vi "Untitled 2.vi"() -> ()   [LabVIEW 2014]
uses:
  <vilib>/vision/NI_Vision_Development_Module.lvlib
  <vilib>/Utility/inputDevices.llb/keyboardAcquire.vi
panel:
  in  "填入飽和磁場分量尖點座標":dbl[][](array[numeric])
  in  "Stop Button":bool
  out "0. 原始畫面":T1(plugin-control)
  in  "1. 範圍選擇":T2={"色相（H）"={0, 255}, "飽和度（S）"={0, 255}, "亮度（L）"={0, 255}} {"亮度（L）" scale=0.0..255.0; "飽和度（S）" scale=0.0..255.0; "色相（H）" scale=0.0..255.0}
  in  "3. Number of Erosion":i32=10
  out "Number of Particles":i32
  out "output cluster":cluster{"X":dbl, "Y":dbl}
  in  "顏色範圍初始化":bool
  in  "Tab Control":T3(tab)
  out "1. 顏色選取":T1(plugin-control)
  out "2. 填補空隙":T1(plugin-control)
  out "3. 移除雜點":T1(plugin-control)
  out "4. 形狀修正":T1(plugin-control)
  out "5. 選取結果":T1(plugin-control)
  out "Particle Measurements":dbl[][](array[numeric])
  out "Error Out":errorcluster
  out "瞬間尖點座標":dbl[][](array[numeric])
  in  "停止":bool
  out "滑鼠位置顏色":T4
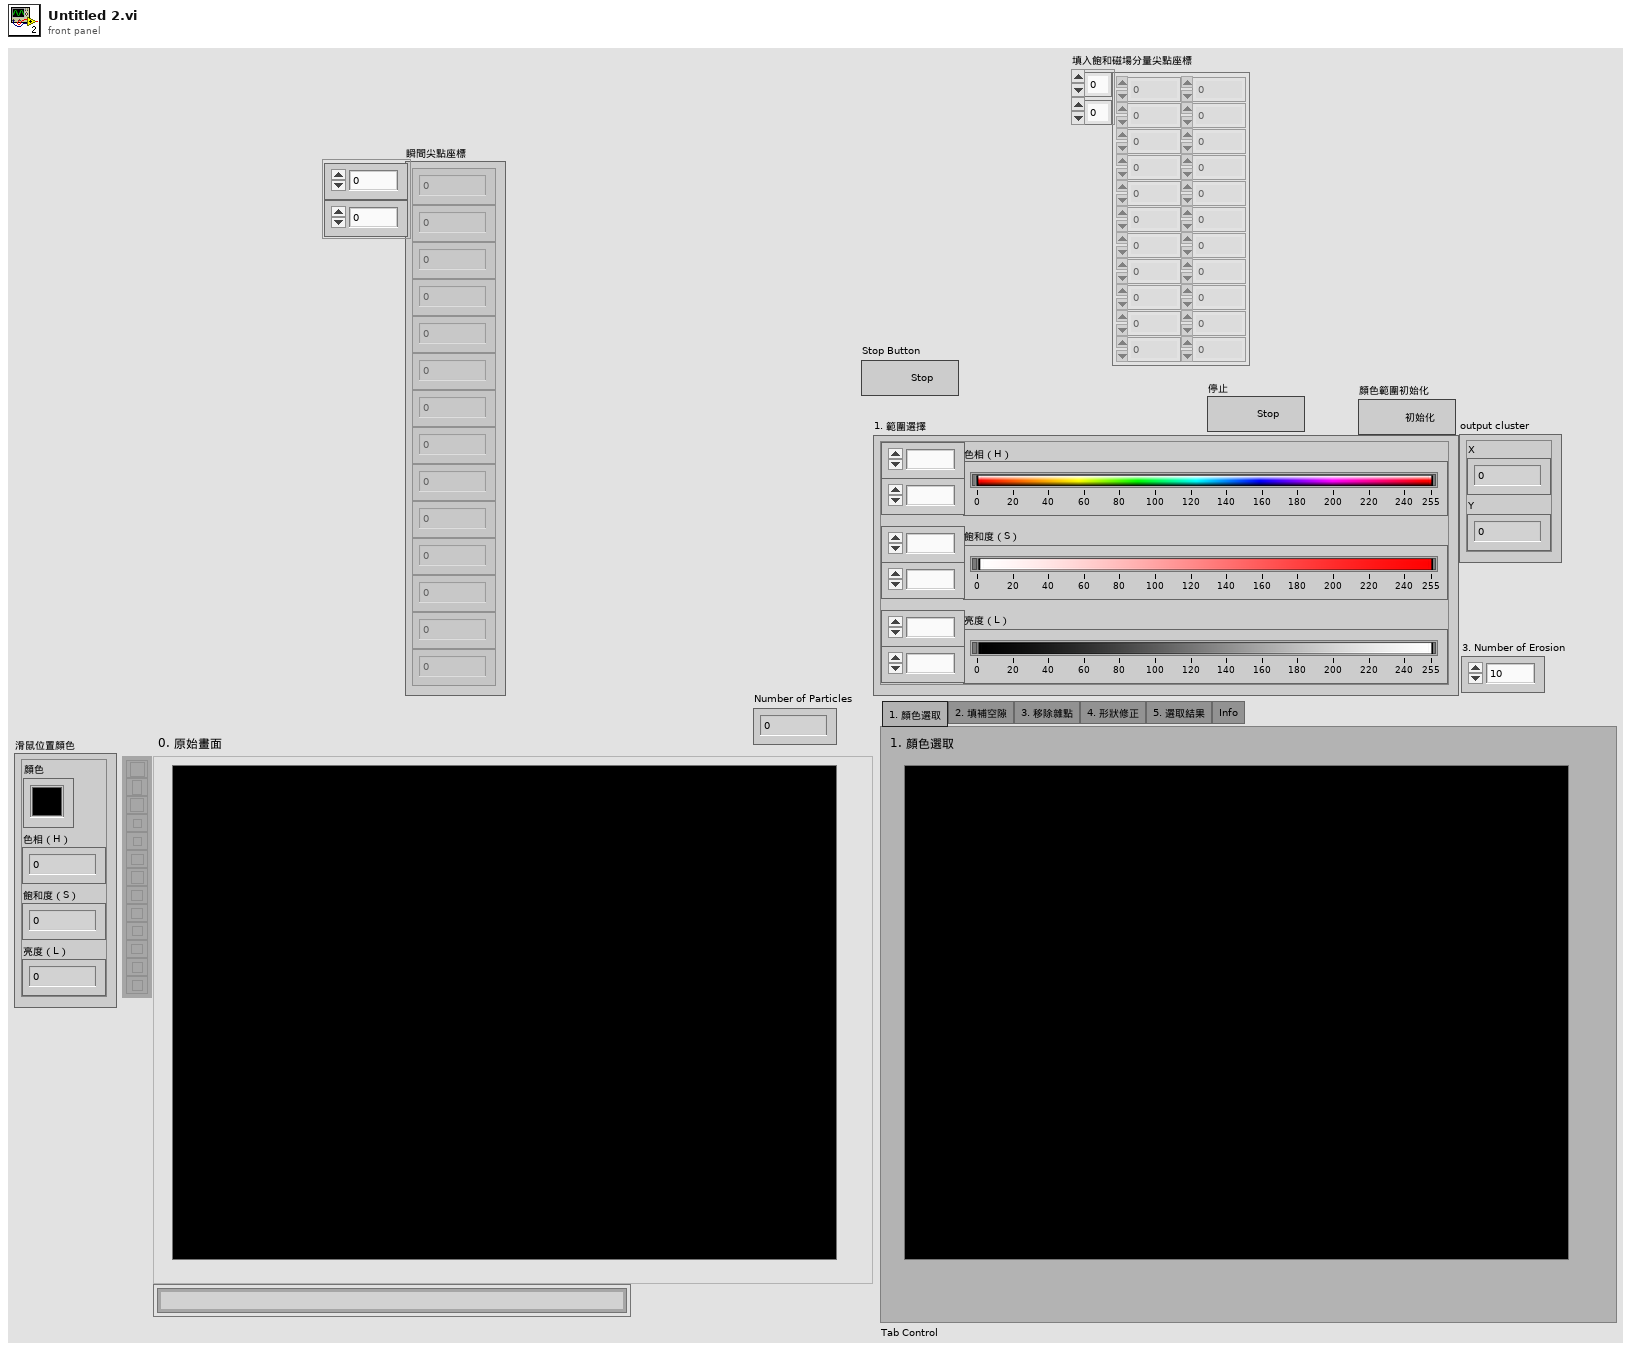
[diagram p1: front panel]
types:
  T1 = typedef "IMAQ Image.ctl" = refnum<image>
  T2 = cluster{"色相（H）":cluster{u8, u8}, "飽和度（S）":cluster{u8, u8}, "亮度（L）":cluster{u8, u8}}
  T3 = enum32{"1. 顏色選取", "2. 填補空隙", "3. 移除雜點", "4. 形狀修正", "5. 選取結果", "Info"}
  T4 = cluster{"色相（H）":u8, "飽和度（S）":u8, "亮度（L）":u8, "顏色":u32}
  T5 = enum16{"0", "1", "2", "3", "4", "5", "6", "7", "8", "9", "A", "B", "C", "D", "E", "F", "G", "H", "I", "J", "K", "L", "M", "N", "O", "P", "Q", "R", "S", "T", "U", "V", "W", "X", "Y", "Z", "F1", "F2", "F3", "F4", "F5", "F6", "F7", "F8", "F9", "F10", "F11", "F12", "F13", "F14", "F15", "ADD", "BACK", "BACKSLASH", "CAPITAL", "COMMA", "DECIMAL", "DELETE", "DIVIDE", "DOWN", "END", "EQUALS", "ESCAPE", "GRAVE (`)", "HOME", "INSERT", "LBRACKET", "LCONTROL", "LEFT", "L ALT", "LSHIFT", "LWIN", "MINUS", "MULTIPLY", "NEXT", "NUMLOCK", "NUMPAD_0", "NUMPAD_1", "NUMPAD_2", "NUMPAD_3", "NUMPAD_4", "NUMPAD_5", "NUMPAD_6", "NUMPAD_7", "NUMPAD_8", "NUMPAD_9", "PAUSE", "PERIOD", "PRIOR (PG UP)", "RBRACKET", "RCONTROL", "RETURN", "RIGHT", "R ALT", "RSHIFT", "RWIN", "SCROLL", "SEMICOLON", "SLASH", "SPACE", "SUBTRACT", "TAB", "UP", "ENTER (num pad)", "' (quote)"}[]
  T6 = enum16{"0", "1", "2", "3", "4", "5", "6", "7", "8", "9", "A", "B", "C", "D", "E", "F", "G", "H", "I", "J", "K", "L", "M", "N", "O", "P", "Q", "R", "S", "T", "U", "V", "W", "X", "Y", "Z", "F1", "F2", "F3", "F4", "F5", "F6", "F7", "F8", "F9", "F10", "F11", "F12", "F13", "F14", "F15", "ADD", "BACK", "BACKSLASH", "CAPITAL", "COMMA", "DECIMAL", "DELETE", "DIVIDE", "DOWN", "END", "EQUALS", "ESCAPE", "GRAVE (`)", "HOME", "INSERT", "LBRACKET", "LCONTROL", "LEFT", "L ALT", "LSHIFT", "LWIN", "MINUS", "MULTIPLY", "NEXT", "NUMLOCK", "NUMPAD_0", "NUMPAD_1", "NUMPAD_2", "NUMPAD_3", "NUMPAD_4", "NUMPAD_5", "NUMPAD_6", "NUMPAD_7", "NUMPAD_8", "NUMPAD_9", "PAUSE", "PERIOD", "PRIOR (PG UP)", "RBRACKET", "RCONTROL", "RETURN", "RIGHT", "R ALT", "RSHIFT", "RWIN", "SCROLL", "SEMICOLON", "SLASH", "SPACE", "SUBTRACT", "TAB", "UP", "ENTER (num pad)", "' (quote)"}
  T7 = cluster{"Numeric":dbl, "Numeric":dbl, "Numeric":dbl, "Numeric":dbl}
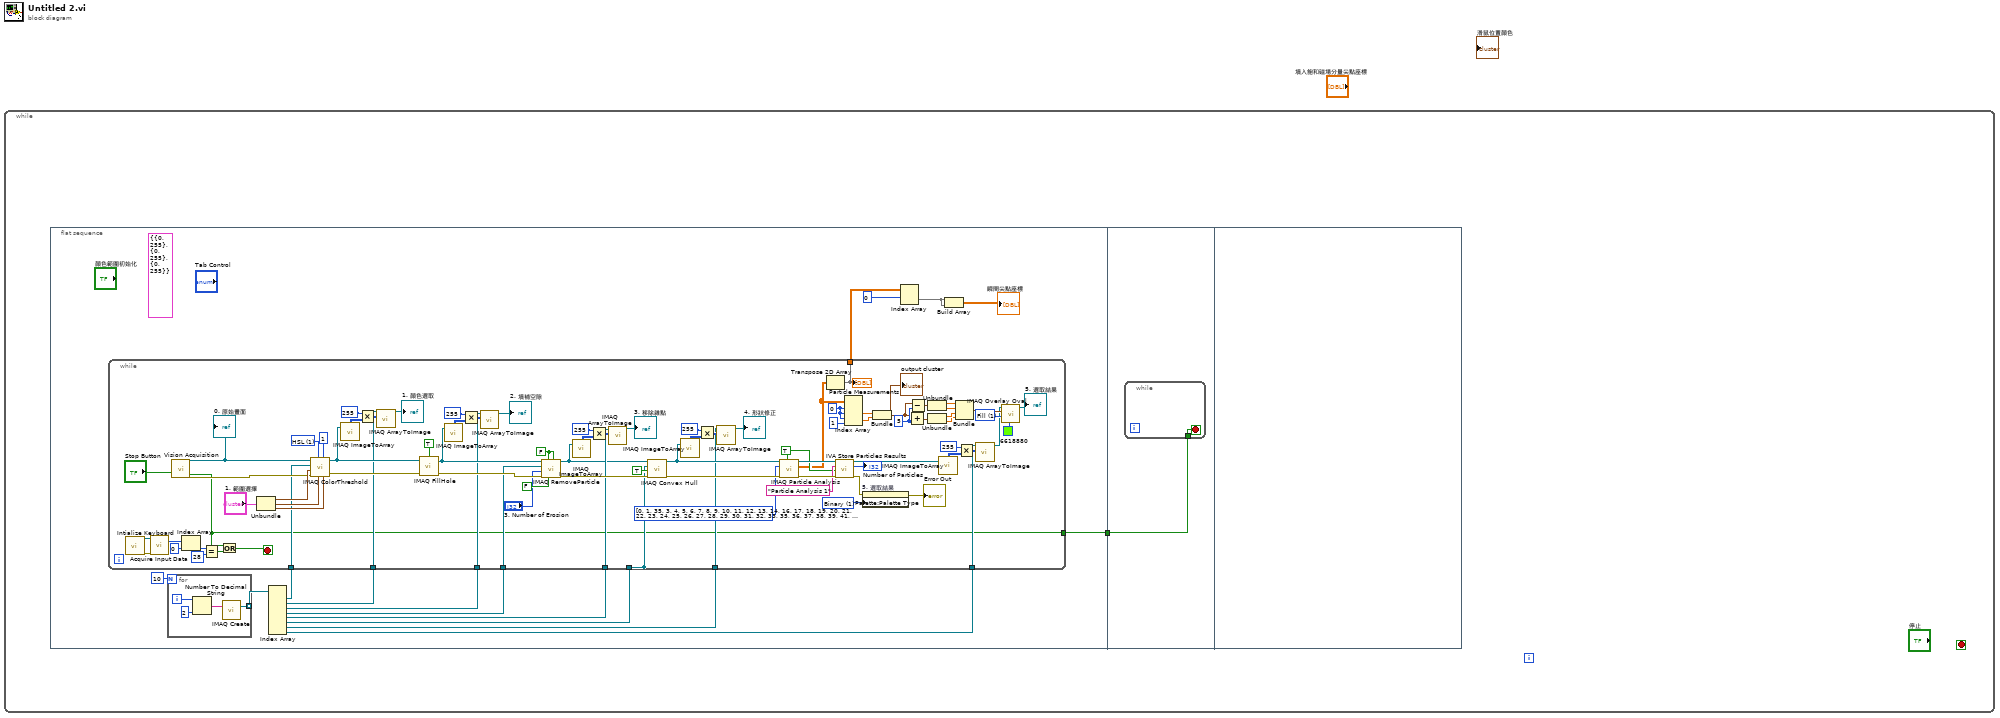
[diagram p0: block diagram]
diagram:
  n1 = while {
    stop <- _ stop-if-true
    n2 = flat-sequence {
      tunnel: [w2] -> w1
      tunnel: w1 -> [w108]
      frame #0 {
        (unwired) T2 {"色相（H）"={0, 255}, "飽和度（S）"={0, 255}, "亮度（L）"={0, 255}} ("範圍選擇")
        n3 = for {
          N: 10 -> [_]
          tunnel: [w17] -> w16 mode=indexing
          i -> [w19]
          n4 = Number To Decimal String(number=w19, width (-)=2) -> (decimal integer string=w18:string)
          n5 = call "IMAQ Create"("Image Name"=w18) -> ("New Image"=w17:T1)  [unwired: 4 in, 1 out]
        }
        n6 = Index Array(array=w16) -> (element #1=w15:T1, element #2=w14:T1, element #3=w13:T1, element #4=w11:T1, element #5=w10:T1, element #6=w9:T1, element #7=w8:T1, element #8=w7:T1)  [unwired: 8 in]
        n7 = while {
          tunnel: w13 -> [w62]
          tunnel: w11 -> [w77]
          tunnel: w9 -> [w75]
          tunnel: [w75] -> _
          tunnel: w14 -> [w69]
          tunnel: w15 -> [w61]
          tunnel: w10 -> [w57]
          tunnel: w8 -> [w49]
          tunnel: w7 -> [w27]
          tunnel: [w24] -> w5
          tunnel: [w21] -> w2
          stop <- w22 stop-if-true
          w32 = u32 1 items=["Frame", "Fill"] ("Drawing Mode (Frame)")
          w41 = 5
          w46 = 0
          w78 = u32 1 items=["Grayscale", "Binary", "Gradient", "Rainbow", "Temperature", "User Defined"] ("Palette")
          w87 = i32[] [0, 1, 35, 3, 4, 5, 6, 7, 8, 9, 10, 11, 12, 13, 14, 16, 17, 18, 19, 20, 21, 22, 23, 24, 25, 26, 27, 28, 29, 30, 31, 32, 33, 35, 36, 37, 38, 39, 41, 42, 43, 45, 46, 48, 49, 50, 51, 53, 54, 55, 56, 58, 59, 60, 61, 62, 63, 64, 65, 66, 68, 69, 70, 71, 72, 73, 74, 75, 76, 77, 78, 79, 80, 81, 82, 83, 84, 85, 86, 87, 88] items=["Center of Mass X", "Center of Mass Y", "First Pixel X", "First Pixel Y", "Bounding Rect Left", "Bounding Rect Top", "Bounding Rect Right", "Bounding Rect Bottom", "Max Feret Diameter Start X", "Max Feret Diameter Start Y", "Max Feret Diameter End X", "Max Feret Diameter End Y", "Max Horiz. Segment Length Left", "Max Horiz. Segment Length Right", "Max Horiz. Segment Length Row", "-", "Bounding Rect Width", "Bounding Rect Height", "Bounding Rect Diagonal", "Perimeter", "Convex Hull Perimeter", "Holes' Perimeter", "Max Feret Diameter", "Equivalent Ellipse Major Axis", "Equivalent Ellipse Minor Axis", "Equivalent Ellipse Minor Axis (Feret)", "Equivalent Rect Long Side", "Equivalent Rect Short Side", "Equivalent Rect Diagonal", "Equivalent Rect Short Side (Feret)", "Average Horiz. Segment Length", "Average Vert. Segment Length", "Hydraulic Radius", "Waddel Disk Diameter", "-", "Area", "Holes' Area", "Particle & Holes' Area", "Convex Hull Area", "Image Area", "-", "Number of Holes", "Number of Horiz. Segments", "Number of Vert. Segments", "-", "Orientation", "Max Feret Diameter Orientation", "-", "% Area/Image Area", "% Area/(Particle & Holes' Area)", "Ratio of Equivalent Ellipse Axes", "Ratio of Equivalent Rect Sides", "-", "Elongation Factor", "Compactness Factor", "Heywood Circularity Factor", "Type Factor", "-", "Sum X", "Sum Y", "Sum XX", "Sum XY", "Sum YY", "Sum XXX", "Sum XXY", "Sum XYY", "Sum YYY", "-", "Moment of Inertia XX", "Moment of Inertia XY", "Moment of Inertia YY", "Moment of Inertia XXX", "Moment of Inertia XXY", "Moment of Inertia XYY", "Moment of Inertia YYY", "Norm. Moment of Inertia XX", "Norm. Moment of Inertia XY", "Norm. Moment of Inertia YY", "Norm. Moment of Inertia XXX", "Norm. Moment of Inertia XXY", "Norm. Moment of Inertia XYY", "Norm. Moment of Inertia YYY", "Hu Moment 1", "Hu Moment 2", "Hu Moment 3", "Hu Moment 4", "Hu Moment 5", "Hu Moment 6", "Hu Moment 7"] ("Pixel Measurements")
          w89 = TRUE ("Connectivity 4/8 (8)")
          w68 = FALSE ("Connectivity 4/8 (8)")
          w98 = u16 1 items=["RGB", "HSL", "HSV", "HSI"] ("Color Mode")
          n8 = call <vilib>:"Intialize Keyboard.vi"() -> ("error out"=w102:errorcluster, "device ID"=w103:refnum<k1>)  [unwired: 10 in]
          n9 = call-poly <vilib>:"Acquire Input Data.vi"("device ID"=w103, "error in (no error)"=w102) -> ("keys pressed"=w104:T5)  [unwired: 15 in, 2 out]
          n10 = call "Vision Acquisition"("Stop (F)"="Stop Button") -> ("Image Out"=w100:T1, "Stopped"=w21:bool, "error out"=w93:errorcluster)  [unwired: 24 in]
          "0. 原始畫面" <- w100
          n11 = Index Array(array=w104, index=0) -> (element=w107:T6)
          n12 = Equal?(x=w107, y=28) -> (x = y?=w101:bool)
          n13 = Or(x=w21, y=w101) -> (x .or. y?=w22:bool)
          n14 = Unbundle("1. 範圍選擇") -> ("色相（H）"=w97:cluster{u8, u8}, "飽和度（S）"=w96:cluster{u8, u8}, "亮度（L）"=w95:cluster{u8, u8})
          n15 = call "IMAQ ColorThreshold"("Blue or Luma or Val or Inten Range"=w95, "Replace Value"=1, "Green or Sat Range"=w96, "Color Mode"=w98, "error in (no error)"=w93, "Red or Hue Range"=w97, "Image Dst"=w61, "Image Src"=w100) -> ("error out"=w80:errorcluster, "Image Dst Out"=w74:T1)  [unwired: 2 out]
          n16 = call "IMAQ ImageToArray"("Image"=w74) -> ("Image Pixels (U8)"=w72:u8[][])  [unwired: 3 in, 4 out]
          n17 = Multiply(x=255, y=w72) -> (x*y=w71:i32[][])
          n18 = call "IMAQ ArrayToImage"("Image Pixels (U8)"=w71, "Image"=w69) -> ("Image Out"=→"1. 顏色選取":T1)  [unwired: 8 in, 1 out]
          n19 = call "IMAQ FillHole"("error in (no error)"=w80, "Image Src"=w74, "Connectivity 4/8 (8)"=TRUE) -> ("error out"=w84:errorcluster, "Image Dst Out"=w63:T1)  [unwired: 1 in, 2 out]
          n20 = call "IMAQ ImageToArray"("Image"=w63) -> ("Image Pixels (U8)"=w66:u8[][])  [unwired: 3 in, 4 out]
          n21 = Multiply(x=255, y=w66) -> (x*y=w67:i32[][])
          n22 = call "IMAQ ArrayToImage"("Image Pixels (U8)"=w67, "Image"=w62) -> ("Image Out"=→"2. 填補空隙":T1)  [unwired: 8 in, 1 out]
          n23 = call "IMAQ RemoveParticle"("Connectivity 4/8 (8)"=w68, "Low Pass/High Pass (Low)"=FALSE, "Square/Hexa (Square)"=w68, "error in (no error)"=w84, "Number of Erosion"="3. Number of Erosion", "Image Dst"=w77, "Image Src"=w63) -> ("error out"=w85:errorcluster, "Image Dst Out"=w55:T1)  [unwired: 3 out]
          n24 = call "IMAQ ImageToArray"("Image"=w55) -> ("Image Pixels (U8)"=w59:u8[][])  [unwired: 3 in, 4 out]
          n25 = Multiply(x=255, y=w59) -> (x*y=w58:i32[][])
          n26 = call "IMAQ ArrayToImage"("Image Pixels (U8)"=w58, "Image"=w57) -> ("Image Out"=→"3. 移除雜點":T1)  [unwired: 8 in, 1 out]
          n27 = call "IMAQ Convex Hull"("error in (no error)"=w85, "Connectivity 4/8 (8)"=TRUE, "Image Dst"=w75, "Image Src"=w55) -> ("error out"=w88:errorcluster, "Image Dst Out"=w50:T1)  [unwired: 6 out]
          n28 = call "IMAQ ImageToArray"("Image"=w50) -> ("Image Pixels (U8)"=w53:u8[][])  [unwired: 3 in, 4 out]
          n29 = Multiply(x=255, y=w53) -> (x*y=w54:i32[][])
          n30 = call "IMAQ ArrayToImage"("Image Pixels (U8)"=w54, "Image"=w49) -> ("Image Out"=→"4. 形狀修正":T1)  [unwired: 8 in, 1 out]
          n31 = call "IMAQ Particle Analysis"("Connectivity 4/8 (8)"=w89, "error in (no error)"=w88, "Pixel Measurements"=w87, "Image"=w50) -> ("error out"=w92:errorcluster, "Particle Measurements (Pixels)"=w47:dbl[][], "Image Out (duplicate)"=w90:T1)  [unwired: 1 in, 4 out]
          n32 = Transpose 2D Array(2D array=w47) -> (transposed array=w24:dbl[][])
          "Particle Measurements" <- w24
          n33 = call <vilib>:"IVA Store Particles Results.vi"("error in (no error)"=w92, "Connectivity 4/8 (8)"=w89, "Step Name"="Particle Analysis 1", "Image in"=w90) -> ("error out"=w79:errorcluster, "Number of Particles"=→"Number of Particles":i32, "Image dup"=w31:T1)  [unwired: 5 out]
          n34 = Index Array(array=w47, index (row) #1=w46, index (col) #1=w46, index (row) #2=w46, index (col) #2=1) -> (element #1=w44:dbl, element #2=w43:dbl)
          n35 = property on="5. 選取結果" class="ImageControl"(error in=w79, "Palette:Palette Type"=w78) -> (error out=→"Error Out":errorcluster)  [unwired: 1 in, 1 out]
          n36 = Bundle("Numeric"=w44, "Numeric"=w43) -> (w40:cluster{"Numeric":dbl, "Numeric":dbl})  [unwired: 1 in]
          "output cluster" <- w40
          n37 = Add(x=w40, y=w41) -> (x+y=w38:cluster{"Numeric":dbl, "Numeric":dbl})
          n38 = Subtract(x=w40, y=w41) -> (x-y=w39:cluster{"Numeric":dbl, "Numeric":dbl})
          n39 = Unbundle(w39) -> ("Numeric"=w37:dbl, "Numeric"=w36:dbl)
          n40 = Unbundle(w38) -> ("Numeric"=w35:dbl, "Numeric"=w34:dbl)
          n41 = call "IMAQ ImageToArray"("Image"=w31) -> ("Image Pixels (U8)"=w28:u8[][])  [unwired: 3 in, 4 out]
          n42 = Bundle("Numeric"=w37, "Numeric"=w36, "Numeric"=w35, "Numeric"=w34) -> (w33:T7)  [unwired: 1 in]
          n43 = Multiply(x=255, y=w28) -> (x*y=w29:i32[][])
          n44 = call "IMAQ ArrayToImage"("Image Pixels (U8)"=w29, "Image"=w27) -> ("Image Out"=w26:T1)  [unwired: 8 in, 1 out]
          n45 = call "IMAQ Overlay Oval"("Color"=u32 6618880, "Drawing Mode (Frame)"=w32, "Bounding Rectangle"=w33, "Image"=w26) -> ("Image Out"=→"5. 選取結果":T1)  [unwired: 6 in, 1 out]
        }
        n46 = Index Array(array=w5, index (row)=0) -> (element=w4:dbl[])  [unwired: 1 in]
        n47 = Build Array(w4, w4) -> (→"瞬間尖點座標":dbl[][])
      }
      frame #1 {
        n48 = while {
          tunnel: w108 -> [w109]
          stop <- w109 stop-if-true
        }
      }
      frame #2 {
      }
    }
  }
